vi "mS Timer.vi"(8 "Error In":errorcluster, 11 "Delay(S)":dbl=0.001 min=1.0 max=10000.0 format="%#_6p") -> (0 "Error Out":errorcluster)   [LabVIEW 2013]
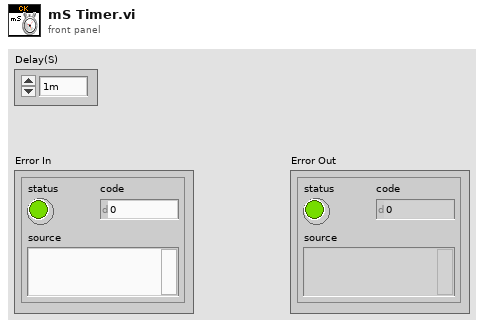
[diagram p1: front panel]
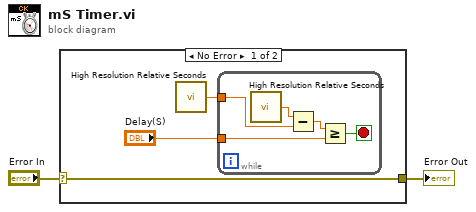
[diagram p0: block diagram]
diagram:
  n1 = case shown="No Error" "Error In" {
    selector: "Error In" -> [w4 w11]
    tunnel: [w4 w11] -> w1
    frame No Error {
      n2 = call <vilib>:"High Resolution Relative Seconds.vi"() -> ("relative seconds"=w5:dbl)
      n3 = while {
        tunnel: w5 -> [w9]
        tunnel: "Delay(S)" -> [w6]
        stop <- w8 stop-if-true
        n4 = call <vilib>:"High Resolution Relative Seconds.vi"() -> ("relative seconds"=w10:dbl)
        n5 = Subtract(x=w10, y=w9) -> (x-y=w7:dbl)
        n6 = Greater Or Equal?(x=w7, y=w6) -> (x >= y?=w8:bool)
      }
    }
    frame Error {
    }
  }
  "Error Out" <- w1
